vi "Linear_Array_StepSize.vi"() -> ()   [LabVIEW 2022 SP3]
panel:
  out "Linear Array":dbl[](array[numeric])
  in  "Step Size":dbl
  in  "Stop":dbl
  in  "Start":dbl
  # "Linear Array Building - Step Size"
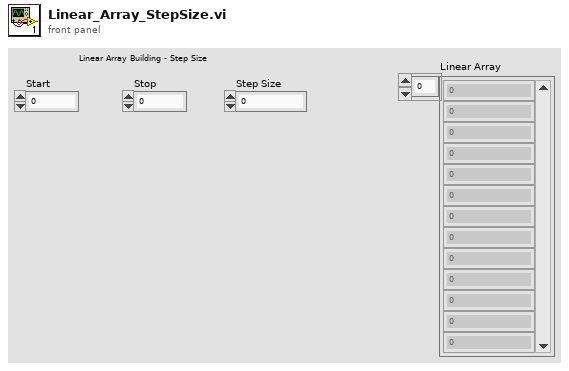
[diagram p1: front panel]
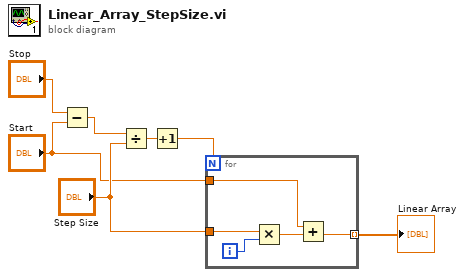
[diagram p0: block diagram]
diagram:
  n1 = Subtract(x="Stop", y="Start") -> (x-y=w6:dbl)
  n2 = Divide(x=w6, y="Step Size") -> (x/y=w5:dbl)
  n3 = Increment(x=w5) -> (x+1=w2:dbl)
  n4 = for {
    N: w2 -> [_]
    tunnel: "Step Size" -> [w11]
    tunnel: [w10] -> w3 mode=indexing
    tunnel: "Start" -> [w8]
    i -> [w12]
    n5 = Multiply(x=w11, y=w12) -> (x*y=w9:dbl)
    n6 = Add(x=w8, y=w9) -> (x+y=w10:dbl)
  }
  "Linear Array" <- w3
